vi "Split.vi"   [LabVIEW 2019, in "xy_utilities.lvlib"]
doc: "Divides <B>XY-Data</B> at <b>index</b> (in units of the x array) and returns <B>XY-Data A</B> and <B>XY-Data B</B>.\n\nThe element at <b>index</b> will be at the beginning of <B>XY-Data B</B>\n\nWire data to the data input to determine the polymorphic instance to use or manually select the instance."
uses:
  xy_utilities.lvlib
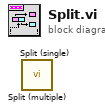
[diagram p0: block diagram]
diagram:
  n1 = call "Split (multiple).vi"() -> ()  [unwired: 9 in, 3 out]
  n2 = call "Split (single).vi"() -> ()  [unwired: 9 in, 3 out]
